vi "fraction.vi"(9 "espesor":dbl, 10 "desnsidad":dbl, 11 "curva atenuation":cluster{"Energia":dbl[], "coeficiente":dbl[]}) -> (3 "Single Plot (X Array and Y Array) 2":cluster{"all rows":dbl[], "all rows":dbl[]}(graph))   [LabVIEW 2021]
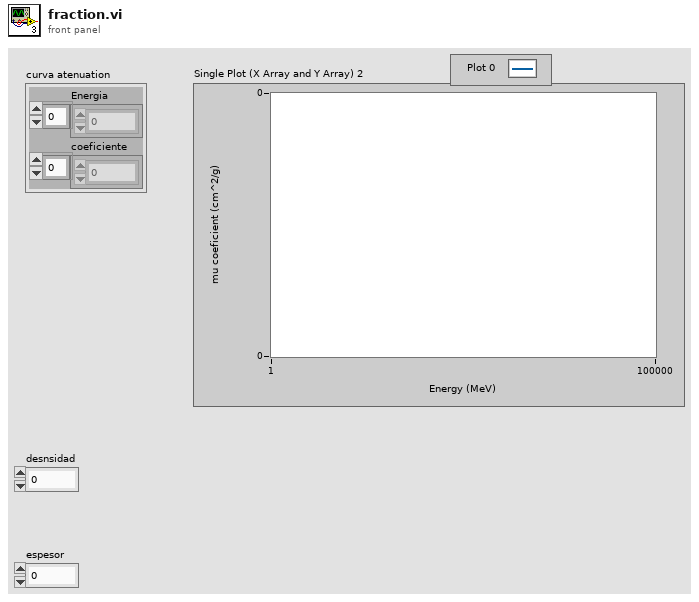
[diagram p1: front panel]
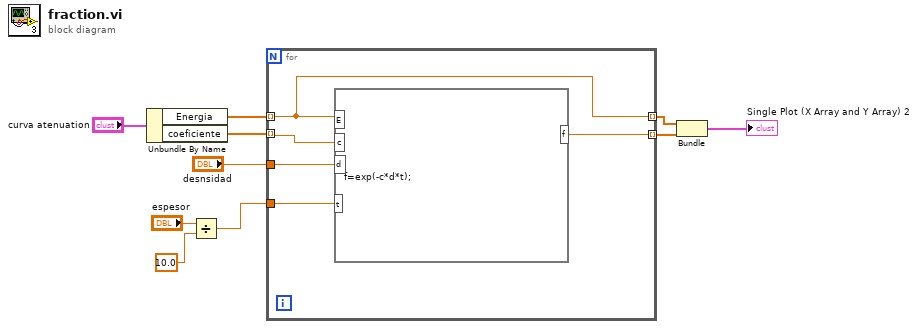
[diagram p0: block diagram]
diagram:
  n1 = Unbundle By Name("curva atenuation") -> ("Energia"=w2:dbl[], "coeficiente"=w3:dbl[])
  n2 = Divide(x="espesor", y=10.0) -> (x/y=w7:dbl)
  n3 = for {
    tunnel: w2 -> [w11] mode=indexing
    tunnel: w3 -> [w15] mode=indexing
    tunnel: "desnsidad" -> [w14]
    tunnel: [w13] -> w8 mode=indexing
    tunnel: w7 -> [w12]
    tunnel: [w11] -> w9 mode=indexing
    n4 = formula code="f=exp(-c*d*t);"("E"=w11, "c"=w15, "d"=w14, "t"=w12) -> ("f"=w13:dbl)
  }
  n5 = Bundle(w9, w8) -> (→"Single Plot (X Array and Y Array) 2":cluster{dbl[], dbl[]})  [unwired: 1 in]
